vi "串口命令输入输出（V1.1）.vi"(0 "VISA resource name":refnum<visa-resource-name> caption="VISA资源名称", 1 "错误输入（无错误）":errorcluster, 2 "string to write":string="*IDN?\r") -> (3 "read string":string caption="读取字符串", 4 "通讯成功":bool, 5 "VISA资源名称输出":refnum<visa-resource-name>, 6 "错误输出":errorcluster)   [LabVIEW 2016]
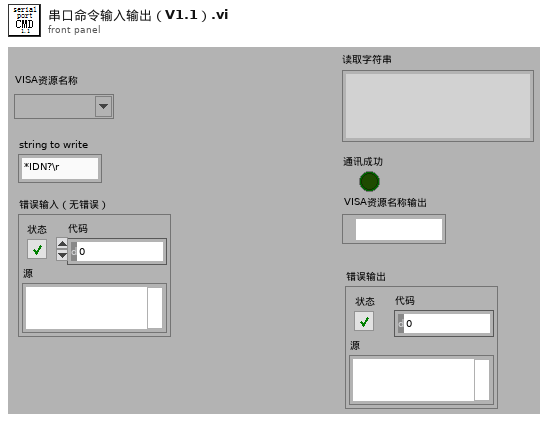
[diagram p1: front panel]
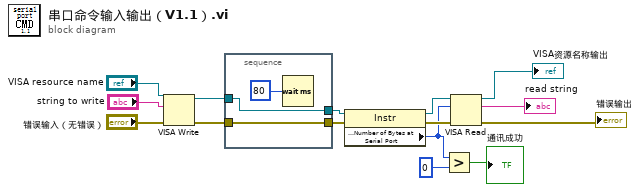
[diagram p0: block diagram]
diagram:
  n1 = VISA Write(VISA resource name="VISA resource name", write buffer="string to write", error in (no error)="错误输入（无错误）") -> (VISA resource name out=w13:refnum<visa-resource-name>, error out=w14:errorcluster)  [unwired: 1 out]
  n2 = stacked-sequence {
    tunnel: w14 -> [w18]
    tunnel: [w18] -> w11
    tunnel: w13 -> [w17]
    tunnel: [w17] -> w12
    frame #0 {
      n3 = Wait (ms)(milliseconds to wait=u32 80 ("读写延时 (ms)")) -> ()  [unwired: 1 out]
    }
  }
  n4 = property class="Instr"(reference=w12, error in=w11) -> (reference out=w10:refnum<visa-resource-name>, error out=w9:errorcluster, "Serial Settings:Number of Bytes at Serial Port"=w7:u32)
  n5 = Greater?(x=w7, y=u32 0) -> (0:→"通讯成功":bool)
  n6 = VISA Read(VISA resource name=w10, byte count=w7, error in (no error)=w9) -> (VISA resource name out=→"VISA资源名称输出":refnum<visa-resource-name>, read buffer=→"read string":string, error out=→"错误输出":errorcluster)  [unwired: 1 out]
